vi "New CSV Logger.vi"(6 "Level":T6, 7 "Logger Name":string, 8 "error in (no error)":errorcluster, 10 "General Options":T2, 11 "File Options":T1) -> (0 "error out":errorcluster)   [LabVIEW 2016, in "Global_logger.lvlib"]
uses:
  Global_logger.lvlib
  Levels.ctl
  General Options.ctl
  Log Fields.ctl
  Level Meaning.ctl
  Sorting.ctl
  File Options.ctl
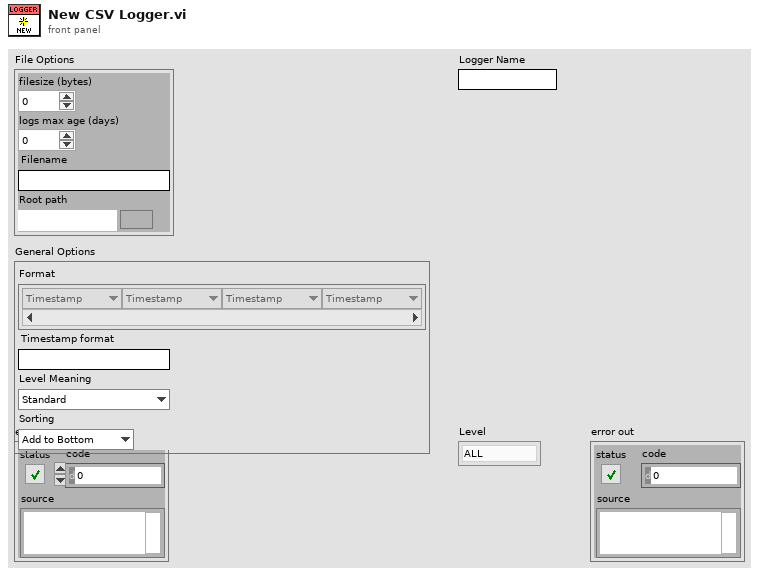
[diagram p1: front panel]
types:
  T1 = typedef "Global_logger.lvlib/File Options.ctl" = cluster{"filesize (bytes)":u32, "logs max age (days) ":i32, "Filename":string, "Root path":path}
  T2 = typedef "Global_logger.lvlib/General Options.ctl" = cluster{"Format":T3[], "Timestamp format":string, "Level Meaning":T4, "Sorting":T5}
  T3 = typedef "Global_logger.lvlib/Log Fields.ctl" = enum16{"Timestamp", "Level", "Message", "Source VI", "Source App", "Logger Name"}
  T4 = typedef "Global_logger.lvlib/Level Meaning.ctl" = enum16{"Standard", "Positive", "Exact"}
  T5 = typedef "Global_logger.lvlib/Sorting.ctl" = enum16{"Add to Bottom", "Add to Top"}
  T6 = typedef "Global_logger.lvlib/Levels.ctl" = enum16{"ALL", "TRACE", "DEBUG", "INFO", "WARN", "ERROR", "FATAL", "OFF"}
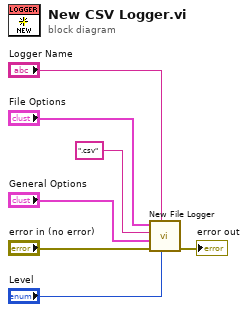
[diagram p0: block diagram]
diagram:
  n1 = call "New File Logger.vi"("Level"="Level", "Logger Name"="Logger Name", "error in (no error)"="error in (no error)", "General Options"="General Options", "Filetype"=".csv", "File Options"="File Options") -> ("error out"=→"error out":errorcluster)  [unwired: 5 in]
